vi "Get Duration of Current State.vi"(10 "samples generated at state":u64, 11 "signal configuration":refnum<class "SV Function.lvclass">) -> (2 "current state duration [s]":dbl, 3 "signal configuration":refnum<class "SV Function.lvclass">)   [LabVIEW 2017, in "SV Function.lvclass"]
uses:
  <vilib>/addons/_NISVFA/_Generation/Signal Generation/SV Function/SV Function.lvclass
  C:/Program Files (x86)/National Instruments/LabVIEW 2017/vi.lib/addons/_NISVFA/_Generation/Signal Generation/SV Signal/SV Signal.lvclass
  <vilib>/addons/_NISVFA/_Generation/Signal Generation/SV Signal/SV Signal.lvclass/SV Signal.ctl
  <vilib>/addons/_NISVFA/_Generation/Signal Generation/SV Signal/Read Ramp-Up.vi
  <vilib>/addons/_NISVFA/_Generation/Signal Generation/SV Signal/Read Ramp-Down.vi
  <vilib>/addons/_NISVFA/_Generation/Signal Generation/SV Signal/Read Transition.vi
  <vilib>/addons/_NISVFA/_Generation/Signal Generation/SV Signal/Read Sample Rate.vi
  <vilib>/addons/_NISVFA/_Generation/Signal Generation/SV Signal/Read Transition Profile.vi
  <vilib>/addons/_NISVFA/_Generation/Signal Generation/SV Signal/Read Generation State.vi
  <vilib>/addons/_NISVFA/_Generation/Signal Generation/SV Signal/Read Post-Measurement Settling Duration.vi
  <vilib>/addons/_NISVFA/_Generation/Signal Generation/SV Signal/Read Measurement Duration.vi
  <vilib>/addons/_NISVFA/_Generation/Signal Generation/SV Signal/Read Pre-Measurement Settling Duration.vi
  <vilib>/addons/_NISVFA/_Generation/Signal Generation/SV Signal/SV Signal.lvclass
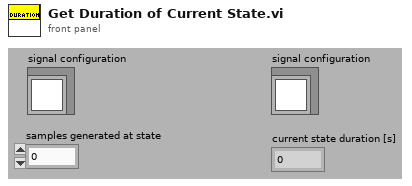
[diagram p1: front panel]
types:
  T1 = typedef "SV Signal.lvclass/sv_Generation State.ctl" = enum16{"Idle", "Ramp Up", "Pre-Measurement Settling", "Measurement", "Post-Measurement Settling", "Discrete Sweep Transition", "Ramp Down", "Update"}
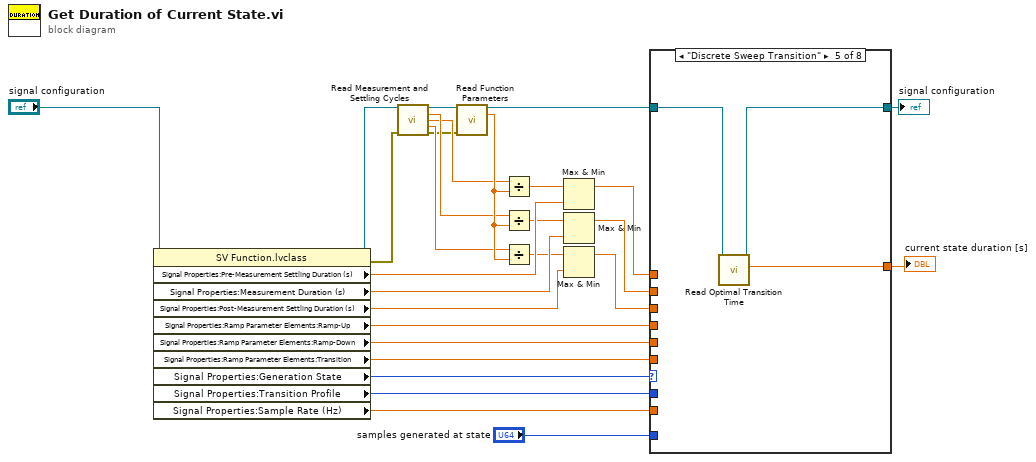
[diagram p0: block diagram]
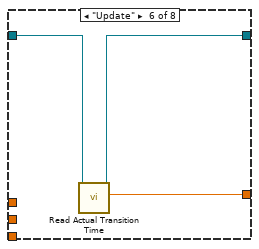
[diagram p7: hidden frame]
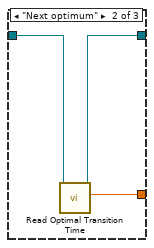
[diagram p9: hidden frame]
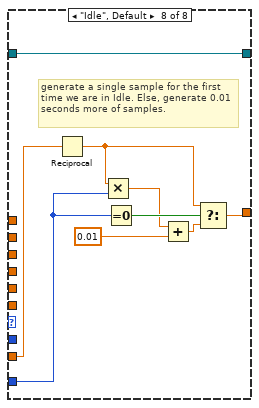
[diagram p11: hidden frame]
diagram:
  n1 = property class="SV Function.lvclass"(reference="signal configuration") -> (reference out=w7:refnum<class "SV Function.lvclass">, error out=w8:errorcluster, "Signal Properties:Pre-Measurement Settling Duration (s)"=w24:dbl, "Signal Properties:Measurement Duration (s)"=w23:dbl, "Signal Properties:Post-Measurement Settling Duration (s)"=w22:dbl, "Signal Properties:Ramp Parameter Elements:Ramp-Up"=w21:dbl, "Signal Properties:Ramp Parameter Elements:Ramp-Down"=w20:dbl, "Signal Properties:Ramp Parameter Elements:Transition"=w19:dbl, "Signal Properties:Generation State"=w18:T1, "Signal Properties:Transition Profile"=w3:enum16{"Immediate", "Next optimum", "Ramp"}, "Signal Properties:Sample Rate (Hz)"=w1:dbl)  [unwired: 1 in]
  n2 = call <vilib>:"Read Measurement and Settling Cycles.vi"("signal configuration"=w7, "error in (no error)"=w8) -> ("signal configuration"=w17:refnum<class "SV Function.lvclass">, "measurement cycles"=w15:dbl, "pre-measurement settling cycles"=w14:dbl, "post-measurement settling cycles"=w13:dbl, "error out"=w9:errorcluster)  [unwired: 9 in]
  n3 = call <vilib>:"Read Function Parameters.vi"("signal configuration"=w17, "error in (no error)"=w9) -> ("signal configuration"=w4:refnum<class "SV Function.lvclass">, "frequency_Hz"=w16:dbl)  [unwired: 8 in, 4 out]
  n4 = Divide(x=w14, y=w16) -> (x/y=w11:dbl)
  n5 = Divide(x=w15, y=w16) -> (x/y=w12:dbl)
  n6 = Divide(x=w13, y=w16) -> (x/y=w10:dbl)
  n7 = Max & Min(x=w11, y=w24) -> (max(x,y)=w26:dbl)  [unwired: 1 out]
  n8 = Max & Min(x=w12, y=w23) -> (max(x,y)=w27:dbl)  [unwired: 1 out]
  n9 = Max & Min(x=w10, y=w22) -> (max(x,y)=w28:dbl)  [unwired: 1 out]
  n10 = case shown="\"Discrete Sweep Transition\"" w18 {
    tunnel: w21 -> [w30 _ _ _ _ _ _ _]
    tunnel: w26 -> [_ w35 _ _ _ _ _ _]
    tunnel: w27 -> [_ _ w37 _ _ _ _ _]
    tunnel: w28 -> [_ _ _ w39 _ _ _ _]
    tunnel: w20 -> [_ _ _ _ _ _ w48 _]
    tunnel: [w29 w35 w37 w39 w42 w45 w47 w59] -> w6
    tunnel: w19 -> [_ _ _ _ _ _ _ _]
    tunnel: [w31 w34 w36 w38 w40 w43 w49 w65] -> w5
    tunnel: w4 -> [w31 w34 w36 w38 w41 w44 w50 w65]
    tunnel: w3 -> [w32 _ _ _ _ _ w46 _]
    tunnel: "samples generated at state" -> [_ _ _ _ _ _ _ w57]
    tunnel: w1 -> [_ _ _ _ _ _ _ w58]
    frame "Ramp Up" {
      n11 = case shown="\"Ramp\"" w32 {
        tunnel: w30 -> [_ w33]
        tunnel: [_ w33] -> w29
        frame "Immediate", Default {
        }
        frame "Ramp" {
        }
      }
    }
    frame "Pre-Measurement Settling" {
    }
    frame "Measurement" {
    }
    frame "Post-Measurement Settling" {
    }
    frame "Discrete Sweep Transition" {
      n12 = call <vilib>:"Read Optimal Transition Time.vi"("signal configuration in"=w41) -> ("optimal transition time"=w42:dbl, "signal configuration out"=w40:refnum<class "SV Function.lvclass">)  [unwired: 8 in, 1 out]
    }
    frame "Update" {
      n13 = call <vilib>:"Read Actual Transition Time.vi"("signal configuration in"=w44) -> ("actual transition time"=w45:dbl, "signal configuration out"=w43:refnum<class "SV Function.lvclass">)  [unwired: 8 in, 1 out]
    }
    frame "Ramp Down" {
      n14 = case shown="\"Immediate\", Default" w46 {
        tunnel: [_ w52 w56] -> w47
        tunnel: w48 -> [_ _ w56]
        tunnel: w50 -> [w51 w54 w55]
        tunnel: [w51 w53 w55] -> w49
        frame "Immediate", Default {
        }
        frame "Next optimum" {
          n15 = call <vilib>:"Read Optimal Transition Time.vi"("signal configuration in"=w54) -> ("optimal transition time"=w52:dbl, "signal configuration out"=w53:refnum<class "SV Function.lvclass">)  [unwired: 8 in, 1 out]
        }
        frame "Ramp" {
        }
      }
    }
    frame "Idle", Default {
      # "generate a single sample for the first time we are in Idle. Else, generate 0.01 seconds more of samples."
      n16 = Reciprocal(x=w58) -> (1/x=w60:dbl)
      n17 = Multiply(x=w60, y=w57) -> (x*y=w62:dbl)
      n18 = Equal To 0?(x=w57) -> (x = 0?=w64:bool)
      n19 = Add(x=w62, y=0.01 ("x")) -> (x+y=w61:dbl)
      n20 = Select(t=w60, s=w64, f=w61) -> (s? t:f=w59:dbl)
    }
  }
  "current state duration [s]" <- w6
  "signal configuration" <- w5
